vi "update_saved_listSD.vi"(1 "error in (no error)":errorcluster, 2 "Numeric":i32, 3 "Experiment":T1, 4 "Experiment in":refnum<class "Experiment.lvclass">) -> (0 "error out":errorcluster)   [LabVIEW 2015]
uses:
  Classes/Experiment.lvclass
  controls/mylistboxRef.ctl
  controls/mylistbox.ctl
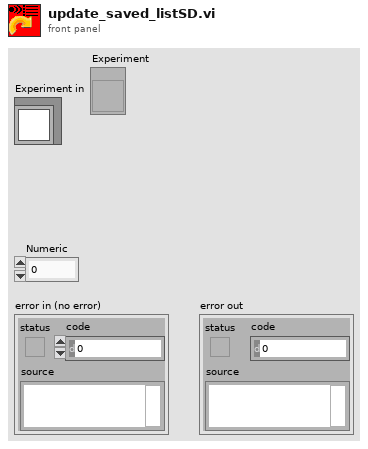
[diagram p1: front panel]
types:
  T1 = typedef "mylistboxRef.ctl" = refnum<vi>
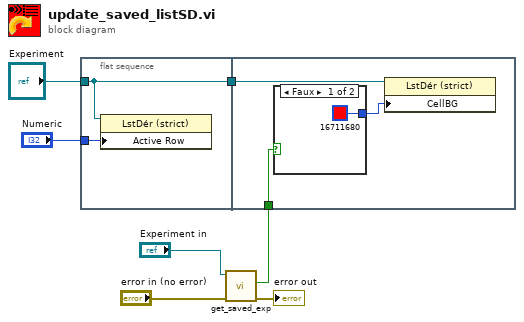
[diagram p0: block diagram]
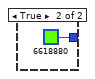
[diagram p2: hidden frame]
diagram:
  n1 = flat-sequence {
    tunnel: "Experiment" -> [w8]
    tunnel: "Numeric" -> [w9]
    tunnel: [w8] -> w7
    tunnel: w7 -> [w12]
    tunnel: w6 -> [w11]
    frame #0 {
      n2 = property on="Property Node" class="LstDér (strict)"(reference=w8, "Active Row"=w9) -> ()  [unwired: 1 in, 2 out]
    }
    frame #1 {
      n3 = case shown="Faux" w11 {
        tunnel: [u32 16711680 u32 6618880] -> w10
        frame False {
        }
        frame True {
        }
      }
      n4 = property on="Property Node" class="LstDér (strict)"(reference=w12, "CellBG"=w10) -> ()  [unwired: 1 in, 2 out]
    }
  }
  n5 = call-dynamic "get_saved_exp.vi"("error in (no error)"="error in (no error)", "Experiment.lvclass in"="Experiment in") -> ("error out"=→"error out":errorcluster, "Saved"=w6:bool)  [unwired: 7 in, 1 out]
